vi "putEnemyDefenseAreaAsObstacleInPotentialField.vi"(4 "multiplier":dbl, 6 "influence radius":dbl, 9 "ArrayOfObstacles in":T1[](array[typedef]), 10 "Game":refnum<class "Game.lvclass">, 11 "Robot":refnum<class "Robot.lvclass">) -> (3 "ArrayOfObstacles out":T1[](array[typedef]))   [LabVIEW 2021, in "Robot.lvclass"]
uses:
  Robot.lvclass
  obstacle.ctl
  D:/RoboIme/horie/SSL_AI/Object_class/Object.lvclass
  Game_class/Game.lvclass
  Object_class/Object.lvclass/Object.ctl
  Game_class/Game.lvclass/Game.ctl
  Field_class/Field.lvclass/Field.ctl
  Field_class/Read enemyGoalPosition.vi
  Game_class/Read FieldRef.vi
  Object_class/Read position(x,y).vi
  <vilib>/Analysis/1siggen.llb/Ramp Pattern by Delta.vi
  Field_class/Field.lvclass
  <vilib>/Analysis/NI_AALBase.lvlib
  Utilities_class/Utilities.lvclass
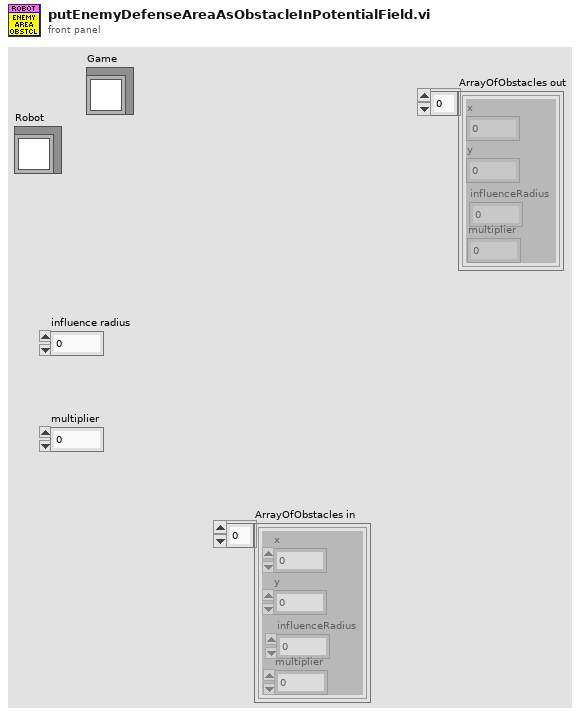
[diagram p1: front panel]
types:
  T1 = typedef "obstacle.ctl" = cluster{"x":dbl, "y":dbl, "influenceRadius":dbl, "multiplier":dbl}
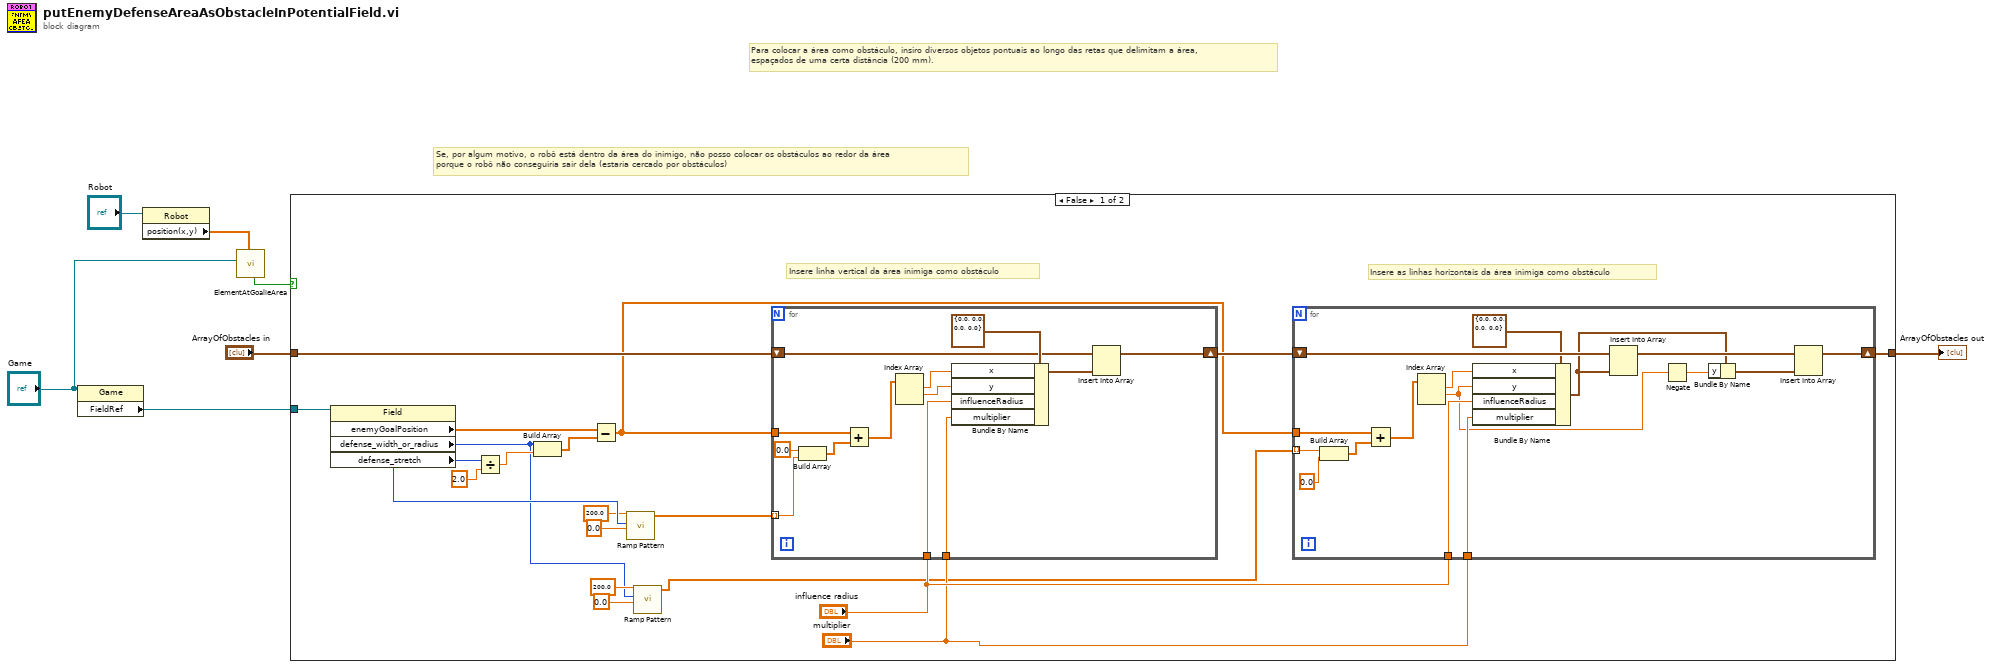
[diagram p0: block diagram]
diagram:
  # "Para colocar a área como obstáculo, insiro diversos objetos pontuais ao longo das retas que delimitam a área,\nespaçados de uma certa distância (200 mm)."
  # "Se, por algum motivo, o robô está dentro da área do inimigo, não posso colocar os obstáculos ao redor da área\nporque o robô não conseguiria sair dela (estaria cercado por obstáculos)"
  n1 = property class="Game"(reference="Game") -> ("FieldRef"=w2:refnum<class "Field.lvclass">)  [unwired: 1 in, 2 out]
  n2 = property class="Robot"(reference="Robot") -> ("position(x,y)"=w4:dbl[])  [unwired: 1 in, 2 out]
  n3 = call "ElementAtGoalieArea.vi"("Elemento pos."=w4, "Game"="Game") -> ("Element at enemy goalkeeper area?"=w3:bool)  [unwired: 5 in, 4 out]
  n4 = case shown="False" w3 {
    tunnel: w2 -> [w26 _]
    tunnel: "ArrayOfObstacles in" -> [w17 w56]
    tunnel: [w15 w56] -> w6
    frame False {
      # "Insere as linhas horizontais da área inimiga como obstáculo"
      # "Insere linha vertical da área inimiga como obstáculo"
      n5 = property class="Field"(reference=w26) -> ("enemyGoalPosition"=w25:dbl[], "defense_width_or_radius"=w9:i32, "defense_stretch"=w20:i32)  [unwired: 1 in, 2 out]
      n6 = Divide(x=w20, y=2.0) -> (x/y=w22:dbl)
      n7 = Build Array(w9, w22) -> (w24:dbl[])
      n8 = Subtract(x=w25, y=w24) -> (x-y=w12:dbl[])
      n9 = call-poly <vilib>:"Ramp Pattern.vi"("start"=0.0, "end"=w20, "delta"=200.0) -> ("Ramp Pattern"=w18:dbl[])  [unwired: 6 in, 2 out]
      n10 = call-poly <vilib>:"Ramp Pattern.vi"("start"=0.0, "end"=w9, "delta"=200.0) -> ("Ramp Pattern"=w8:dbl[])  [unwired: 6 in, 2 out]
      n11 = for {
        tunnel: w18 -> [w48] mode=indexing
        shift-right: [w53] -> w16
        shift-left: w17 -> [w52]
        tunnel: "influence radius" -> [w44]
        tunnel: "multiplier" -> [w43]
        tunnel: w12 -> [w51]
        n12 = Build Array(0.0 ("element"), w48) -> (w50:dbl[])
        n13 = Add(x=w51, y=w50) -> (x+y=w45:dbl[])
        n14 = Index Array(array=w45) -> (element #1=w47:dbl, element #2=w46:dbl)  [unwired: 2 in]
        n15 = Bundle By Name(cluster=T1 {"x"=0.0, "y"=0.0, "influenceRadius"=0.0, "multiplier"=0.0} ("ArrayOfObstacles in 2"), "x"=w47, "y"=w46, "influenceRadius"=w44, "multiplier"=w43) -> (w54:T1)
        n16 = Insert Into Array(array=w52, new element=w54) -> (w53:T1[])  [unwired: 1 in]
      }
      n17 = for {
        shift-right: [w33] -> w15
        shift-left: w16 -> [w42]
        tunnel: "influence radius" -> [w30]
        tunnel: "multiplier" -> [w37]
        tunnel: w8 -> [w35] mode=indexing
        tunnel: w12 -> [w41]
        n18 = Build Array(w35, 0.0 ("element")) -> (w40:dbl[])
        n19 = Add(x=w41, y=w40) -> (x+y=w38:dbl[])
        n20 = Index Array(array=w38) -> (element #1=w39:dbl, element #2=w27:dbl)  [unwired: 2 in]
        n21 = Bundle By Name(cluster=T1 {"x"=0.0, "y"=0.0, "influenceRadius"=0.0, "multiplier"=0.0} ("ArrayOfObstacles in 2"), "x"=w39, "y"=w27, "influenceRadius"=w30, "multiplier"=w37) -> (w29:T1)
        n22 = Insert Into Array(array=w42, new element=w29) -> (w34:T1[])  [unwired: 1 in]
        n23 = Negate(x=w27) -> (-x=w28:dbl)
        n24 = Bundle By Name(cluster=w29, "y"=w28) -> (w31:T1)
        n25 = Insert Into Array(array=w34, new element=w31) -> (w33:T1[])  [unwired: 1 in]
      }
    }
    frame True {
    }
  }
  "ArrayOfObstacles out" <- w6
